vi "3RD_STAGE.vi"() -> (0 "Stage 3 Coolant Temperature":dbl(graph), 1 "Stage 3 Pressure":dbl(graph), 2 "Stage 3 Temperature":dbl(graph), 3 "Stage-III Temperature Transmitter (After Cooler)":dbl, 4 "Stage-III Temperature Transmitter":dbl, 5 "Stage-III Pressure Transmitter":dbl)   [LabVIEW 2014]
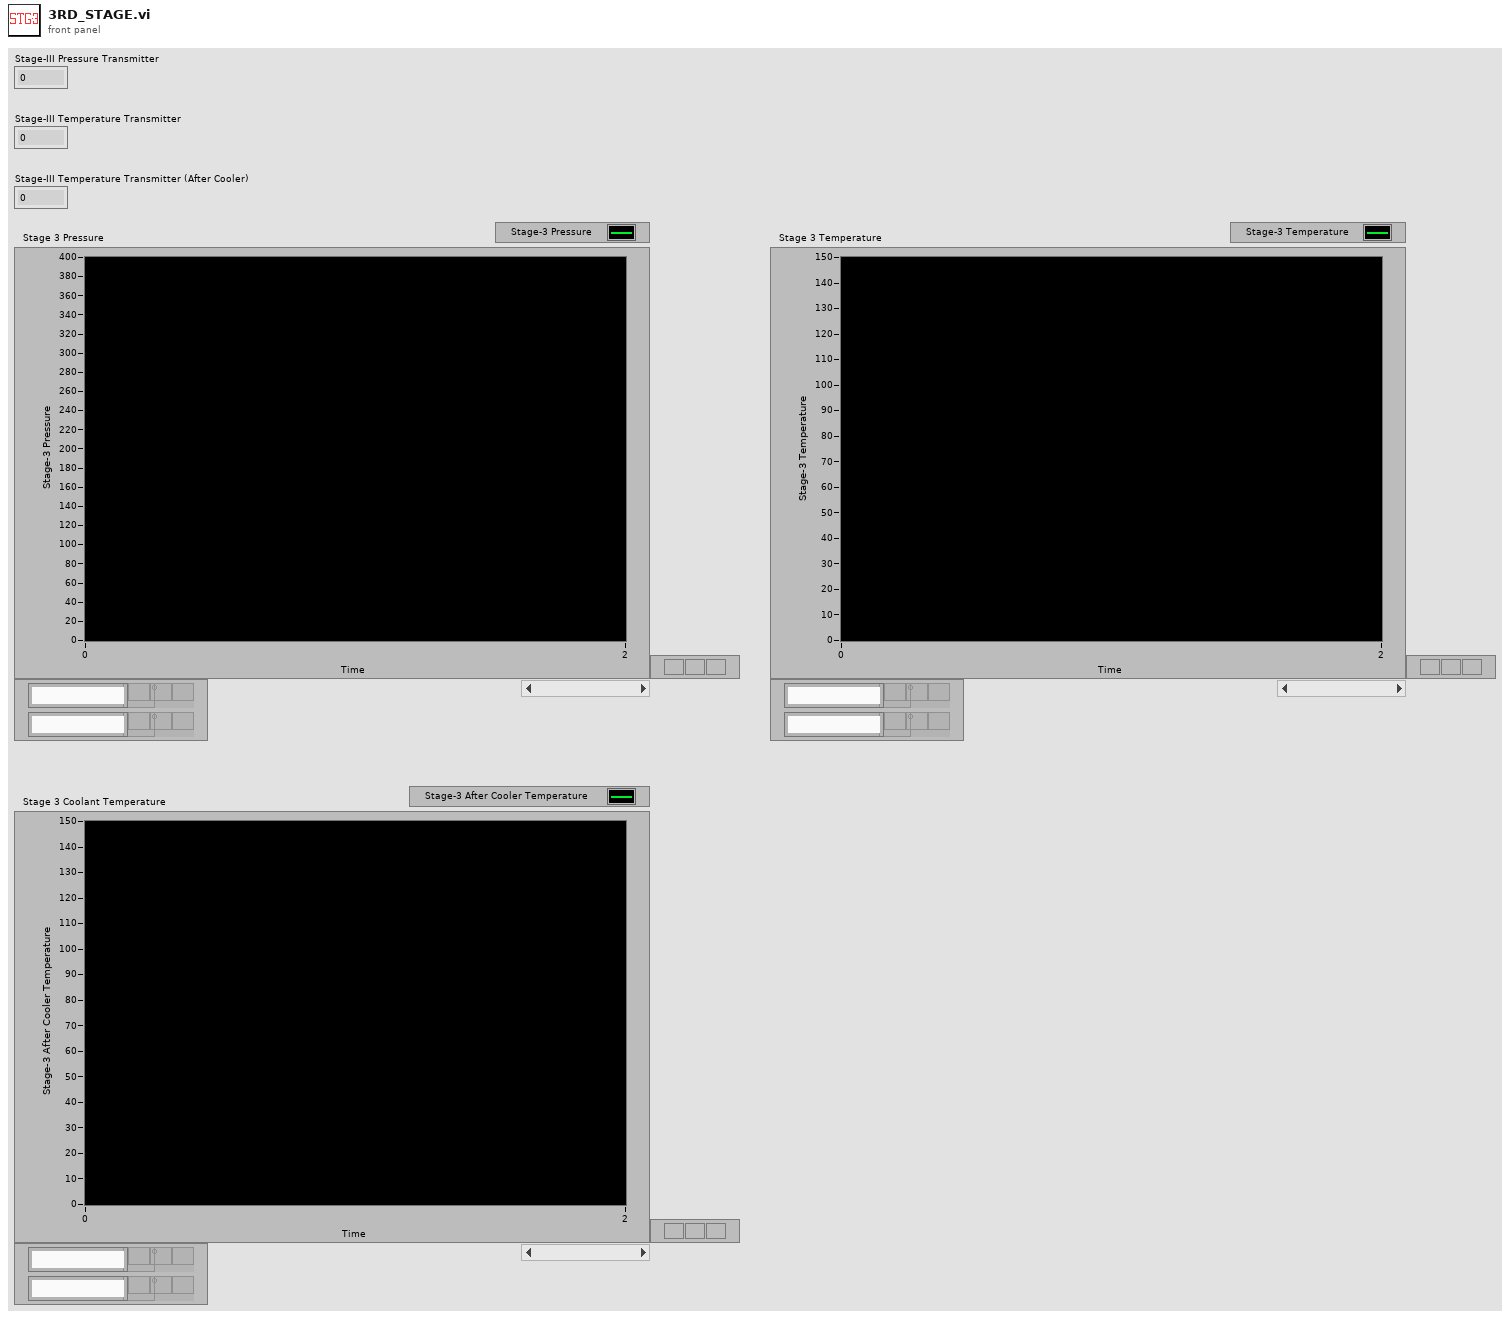
[diagram p1: front panel]
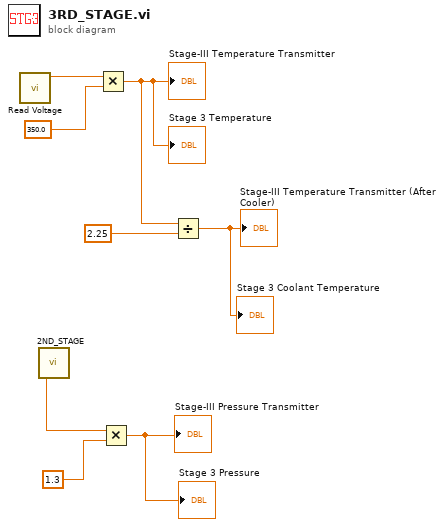
[diagram p0: block diagram]
diagram:
  n1 = call "Read Voltage.vi"() -> ("voltage"=w2:dbl)  [unwired: 6 in, 1 out]
  n2 = call "2ND_STAGE.vi"() -> ("Stage-2 Pressure"=w1:dbl)  [unwired: 5 out]
  n3 = Multiply(x=w2, y=350.0) -> (x*y=w4:dbl)
  "Stage-III Temperature Transmitter" <- w4
  "Stage 3 Temperature" <- w4
  n4 = Multiply(x=w1, y=1.3) -> (x*y=→"Stage-III Pressure Transmitter" →"Stage 3 Pressure":dbl)
  n5 = Divide(x=w4, y=2.25) -> (x/y=→"Stage-III Temperature Transmitter (After Cooler)" →"Stage 3 Coolant Temperature":dbl)
